vi "format string.vi"(11 "Label.Text":string) -> (3 "String":string)   [LabVIEW 2025, in "Tools.lvlib"]
doc: "replaces all spaces with \"_\" and turns all to lower case so e.g. parameter names fit nicely into the python code."
uses:
  Tools.lvlib
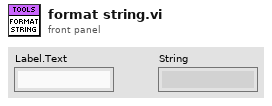
[diagram p1: front panel]
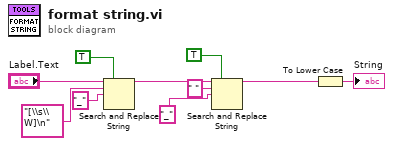
[diagram p0: block diagram]
diagram:
  n1 = Search and Replace String(replace all?=TRUE ("replace all? (F)"), input string="Label.Text", search string="[\\s\\W]\n", replace string="_" ("replace string (\"\")")) -> (result string=w6:string)  [unwired: 4 in, 3 out]
  n2 = Search and Replace String(replace all?=TRUE ("replace all? (F)"), input string=w6, search string=" ", replace string="_" ("replace string (\"\")")) -> (result string=w4:string)  [unwired: 4 in, 3 out]
  n3 = To Lower Case(string=w4) -> (all lower case string=→"String":string)
